vi "TCP Check Connection (By Reference).vi"(8 "error in":errorcluster, 10 "connection in":T3, 11 "connection manager ref in":T2) -> (0 "error out":errorcluster, 1 "disconnected?":bool, 2 "connection out":T3, 3 "connection manager ref out":T2, 4 "properties out":T1)   [LabVIEW 2010, in "NI STM.lvlib"]
doc: "This VI removes the host connection from the connection manager list if it becomes disconnected for any reason.\n\nCopyright 2015, 2016, 2017 National Instruments Corporation\n\nLicensed under the Apache License, Version 2.0 (the \"License\"); you may not use this file except in compliance with the License.\n\n You may obtain a copy of the License at\n\n http://www.apache.org/licenses/LICENSE-2.0\n\nUnless required by applicable law or agreed to in writing, software distributed under the License is distributed on an \"AS IS\" BASIS, WITHOUT WARRANTIES OR CONDITIONS OF ANY KIND, either express or implied.\n\nSee the License for the specific language governing permissions and limitations under the License."
uses:
  NI STM.lvlib
  TCP/TCP Connection Info.ctl
  SubVIs/MetaDataElement.ctl
  TCP Connection Manager Reference.ctl
  TCP Connection Manager State Variables.ctl
  TCP Connection Properties.ctl
  TCP Connection Method.ctl
  SubVIs/Generate STM Error.vi
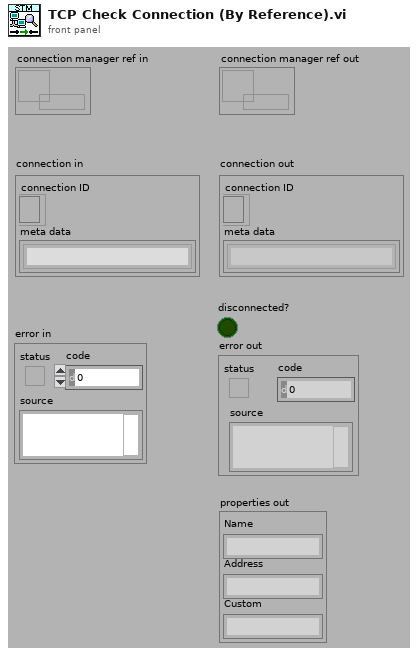
[diagram p1: front panel]
types:
  T1 = typedef "NI STM.lvlib/TCP Connection Properties.ctl" = cluster{"Name":string, "Address":string, "Custom":string}
  T2 = typedef "NI STM.lvlib/TCP Connection Manager Reference.ctl" = refnum<data-value>
  T3 = typedef "NI STM.lvlib/TCP Connection Info.ctl" = cluster{"connection ID":refnum<k5>, "meta data":T4[]}
  T4 = typedef "NI STM.lvlib/MetaDataElement.ctl" = string
  T5 = typedef "NI STM.lvlib/TCP Connection Method.ctl" = enum16{"Initialize", "Add Connection", "Set Properties", "Get Connection(s)", "Remove Connection", "Remove All Connections", "Get Connection Count"}
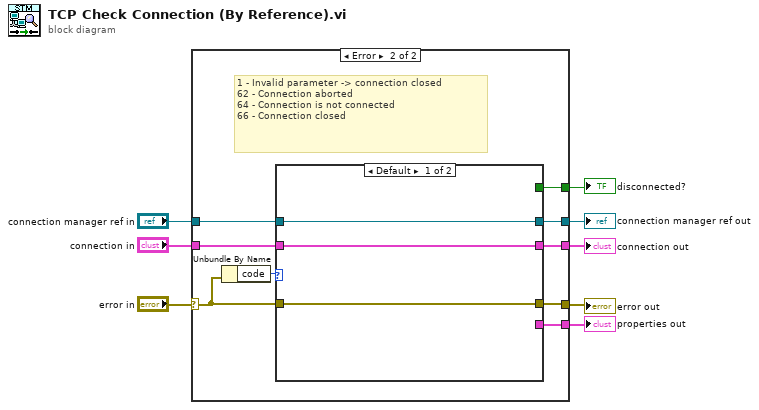
[diagram p0: block diagram]
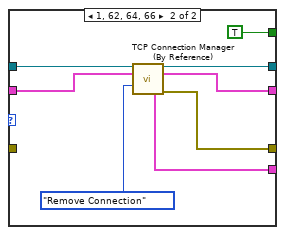
[diagram p3: hidden frame]
diagram:
  n1 = case shown="Error" "error in" {
    selector: "error in" -> [w11 w19]
    tunnel: [w11 w18] -> w7
    tunnel: "connection in" -> [w10 w17]
    tunnel: [w10 w16] -> w5
    tunnel: [_ w15] -> w4
    tunnel: "connection manager ref in" -> [w9 w14]
    tunnel: [w9 w13] -> w2
    tunnel: [_ w12] -> w1
    frame No Error {
    }
    frame Error {
      # "1 - Invalid parameter -> connection closed\n62 - Connection aborted\n64 - Connection is not connected\n66 - Connection closed"
      n2 = Unbundle By Name(w19) -> ("code"=w20:i32)
      n3 = case shown="Default" w20 {
        tunnel: w19 -> [w23 _]
        tunnel: [w23 w29] -> w18
        tunnel: w17 -> [w22 w28]
        tunnel: [w22 w27] -> w16
        tunnel: [_ TRUE] -> w15
        tunnel: w14 -> [w21 w26]
        tunnel: [w21 w25] -> w13
        tunnel: [_ w24] -> w12
        frame Default {
        }
        frame 1, 62, 64, 66 {
          n4 = call "TCP Connection Manager (By Reference).vi"("connection manager ref in"=w26, "connection in"=w28, "method"=TCP_Connection_Method."Remove Connection" ("Method")) -> ("connection manager ref out"=w25:T2, "connection out"=w27:T3, "properties out"=w24:T1, "error out"=w29:errorcluster)  [unwired: 6 in, 3 out]
        }
      }
    }
  }
  "error out" <- w7
  "connection out" <- w5
  "disconnected?" <- w4
  "connection manager ref out" <- w2
  "properties out" <- w1
